vi "GetNewSetName.vi"(9 "Settings":T1={"Name of test"="", "Date"=timestamp(0 s since 1904-01-01), "Location"="", "Template"="", "Soundcard"="", "resolution"=0, "Sampling rate"=0, "Ch1 Gain "=0.0, "Ch2 Gain"=0.0, "Sample time (s)"=0.0, "Pre-trigger (s)"=0.0, "Hammer Threshold"=0.0, "Positions"=0, "Taps/Position"=0, "Set Names"="", "Freq resolution"=0.0, "Hammer cutoff"=0.0, "Mic cutoff"=0.0, "Double bounce "=0.0, "Hammer Cal"=0.0, "dB Offset"=0.0, "Accel Cal"=0.0, "Vibrometer Cal"=0.0, "Mic Cal"=0.0, "Output"=0, "Voltage Cal"=0.0, "Vibrometer Port"="", "Range"=0, "High Pass"=0, "Bandwidth"=0, "X Range"=[], "Y Range"=[], "dB Spread"=0.0, "Trigger"=0, "Ch_1"=25, "Ch_2"=25, "flip?"=FALSE, "60Hz"=FALSE, "Time offset"=0.0, "Piezo Cal"=1.0, "Default Notes"=""} {"Ch_2" min=1 step=1; "Ch_1" min=1 max=100 step=1; "Trigger" items=["Hammer (force)", "Self-tap", "Spacebar"]; "Bandwidth" items=["1 kHz"=1, "5 kHz"=5, "10 kHz"=10, "25 kHz"=25, "50 kHz"=50, "100 kHz"=100]; "High Pass" items=["Off", "13 Hz", "104 Hz"]; "Range" items=["10 mm/s"=1, "20 mm/s"=2, "50 mm/s"=5, "100 mm/s"=10, "200 mm/s"=20, "500 mm/s"=50, "1 m/s"=100, "2 m/s"=200]; "Output" items=["Accelerometer", "Speed (from acceleration)", "Microphone", "Vibrometer", "Piezo"]; "Voltage Cal" format="%#_13g"; "Ch2 Gain" format="%#_13g"; "Ch1 Gain" format="%#_13g"; "Double bounce" min=0.0; "Mic cutoff" min=0.0 format="%#_4g"; "Hammer cutoff" min=0.0 format="%#_4g"; "Freq resolution" min=0.0; "Pre-trigger (s)" format="%#_13g"; "Date" format="%<%H:%M\n%d/%m/%y>T"; "resolution" items=["16 bit"=16, "24 bit"=24, "32 bit"=32]; "Sampling rate" items=["22050 samp/s"=22050, "44100 samp/s"=44100, "48000 samp/s"=48000]}, 11 "Info":cluster{"Set":string, "Position":i32, "Tap":i32}) -> (1 "last tap?":bool, 3 "String":string)   [LabVIEW 2022 SP3]
uses:
  PreferencesControl.ctl
panel:
  out "Location":cluster{"Set":i16, "Position":i16, "Tap":i16}
  # "Hz"
  # "dB"
  # "dB"
  # "sec"
  # "sec"
  # "mV/Pa"
  # "mV/m/s2"
  # "mV/mm/s"
  # "V/N"
  # "sec"
  # "sec"
  # "mV/N"
  # "a.u."
  # "a.u."
  # "sec"
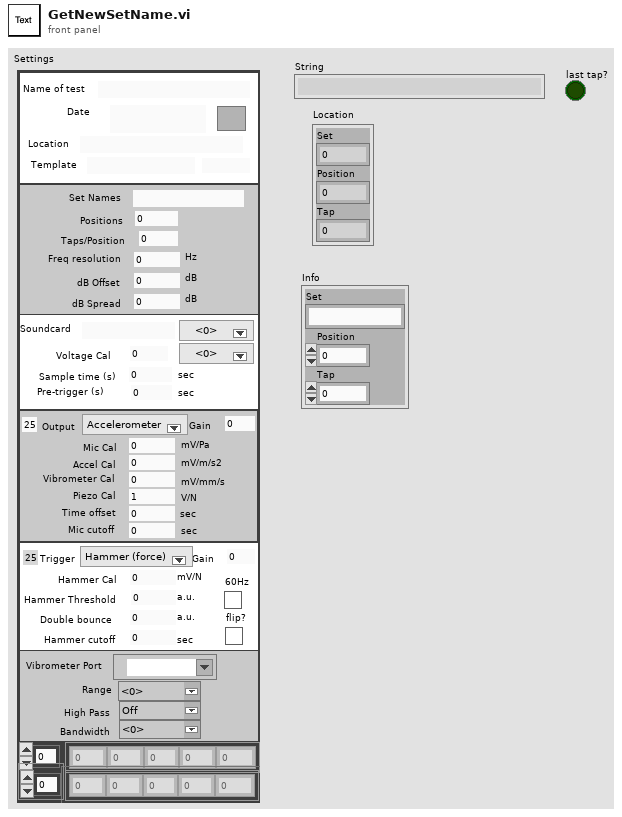
[diagram p1: front panel]
types:
  T1 = typedef "PreferencesControl.ctl" = cluster{"Name of test":string, "Date":timestamp, "Location":string, "Template":string, "Soundcard":string, "resolution":u16, "Sampling rate":u16, "Ch1 Gain ":dbl, "Ch2 Gain":dbl, "Sample time (s)":dbl, "Pre-trigger (s)":dbl, "Hammer Threshold":dbl, "Positions":i16, "Taps/Position":i16, "Set Names":string, "Freq resolution":dbl, "Hammer cutoff":dbl, "Mic cutoff":dbl, "Double bounce ":dbl, "Hammer Cal":dbl, "dB Offset":dbl, "Accel Cal":dbl, "Vibrometer Cal":dbl, "Mic Cal":dbl, "Output":u16, "Voltage Cal":dbl, "Vibrometer Port":refnum<visa-resource-name>, "Range":u16, "High Pass":u16, "Bandwidth":u16, "X Range":cluster{"Minimum":dbl, "Maximum":dbl, "Increment":dbl, "Minor Increment":dbl, "Start":dbl}[], "Y Range":cluster{"Minimum":dbl, "Maximum":dbl, "Increment":dbl, "Minor Increment":dbl, "Start":dbl}[], "dB Spread":dbl, "Trigger":u16, "Ch_1":u8, "Ch_2":u8, "flip?":bool, "60Hz":bool, "Time offset":dbl, "Piezo Cal":dbl, "Default Notes":string}
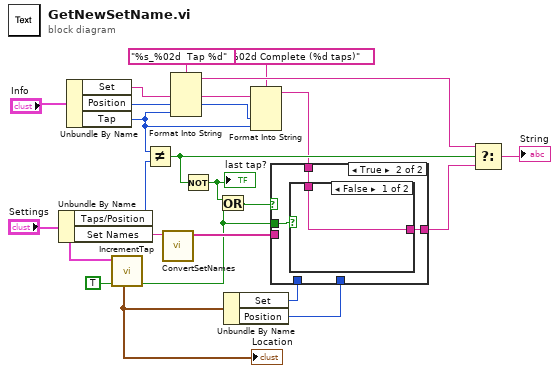
[diagram p0: block diagram]
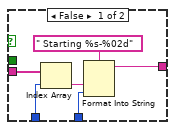
[diagram p2: hidden frame]
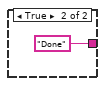
[diagram p3: hidden frame]
diagram:
  n1 = Unbundle By Name("Settings") -> ("Taps/Position"=w13:i16, "Set Names"=w20:string)
  n2 = Unbundle By Name("Info") -> ("Set"=w4:string, "Position"=w3:i32, "Tap"=w1:i32)
  n3 = call "IncrementTap.vi"("Reset?"=TRUE, "Settings"="Settings") -> ("Done?"=w6:bool, "Next Location"=w16:cluster{"Set":i16, "Position":i16, "Tap":i16})  [unwired: 4 in, 4 out]
  "Location" <- w16
  n4 = Not Equal?(x=w1, y=w13) -> (x != y?=w12:bool)
  n5 = call "ConvertSetNames.vi"("Set Names"=w20) -> ("Set Names"=w21:string[])  [unwired: 10 in]
  n6 = Format Into String(format string="%s_%02d  Tap %d", w4, w3, w1) -> (resulting string=w10:string)  [unwired: 2 in, 1 out]
  n7 = Not(x=w12) -> (.not. x?=w8:bool)
  "last tap?" <- w8
  n8 = Or(x=w8, y=w6) -> (x .or. y?=w7:bool)
  n9 = Unbundle By Name(w16) -> ("Set"=w22:i16, "Position"=w17:i16)
  n10 = Format Into String(format string="%s_%02d Complete (%d taps)", w4, w3, w1) -> (resulting string=w2:string)  [unwired: 2 in, 1 out]
  n11 = case shown="True" w7 {
    tunnel: w22 -> [w27 _]
    tunnel: w21 -> [w26 _]
    tunnel: [w25 w31] -> w11
    tunnel: w17 -> [w24 _]
    tunnel: w6 -> [_ w30]
    tunnel: w2 -> [_ w29]
    frame False {
      n12 = Index Array(array=w26, index=w27) -> (element=w28:string)
      n13 = Format Into String(format string=" Starting %s-%02d", w28, w24) -> (resulting string=w25:string)  [unwired: 2 in, 1 out]
    }
    frame True {
      n14 = case shown="False" w30 {
        tunnel: [w32 "Done"] -> w31
        tunnel: w29 -> [w32 _]
        frame False {
        }
        frame True {
        }
      }
    }
  }
  n15 = Select(t=w10, s=w12, f=w11) -> (s? t:f=→"String":string)
